vi "Exercise 4.2.vi"() -> ()   [LabVIEW 2010]
panel:
  out "Loop Iterations":i32
  out "Dispense\nChange":bool
  out "Change\nDispensed ($)":dbl format="%.2f"
  out "Vend\nSoda":bool
  out "Money Inserted ($)":dbl format="%.2g"
  in  "Coin to Insert":T1(ring)
  in  "stop":bool
  in  "Insert Coin":bool
  # "All Products in this vending machine cost $0.50"
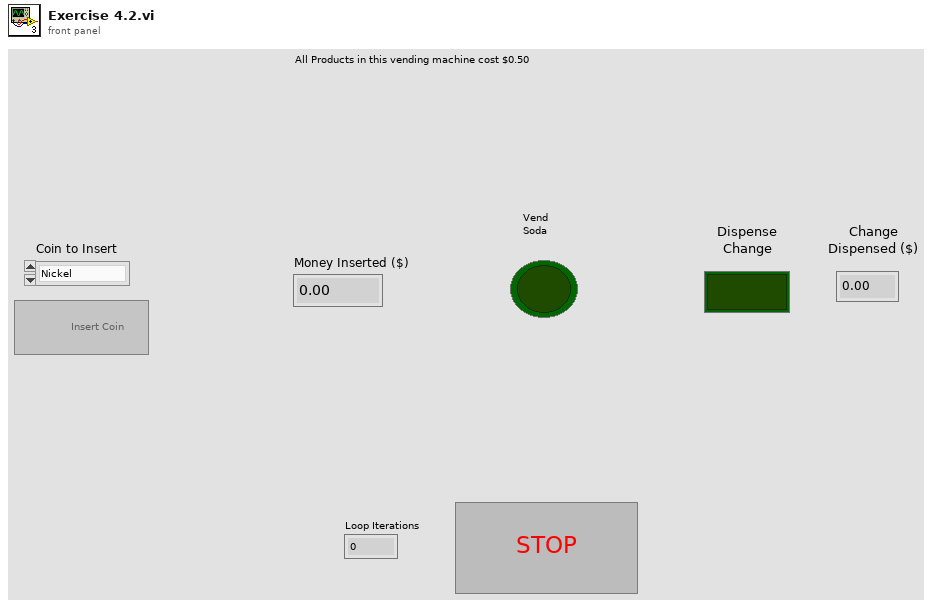
[diagram p1: front panel]
types:
  T1 = enum16{"Nickel", "Dime", "Quarter", "Exit", "Vend", "Change", "Wait", "Initialize"}
  T2 = enum8{"Enabled", "Disabled", "Disabled and Grayed Out"}
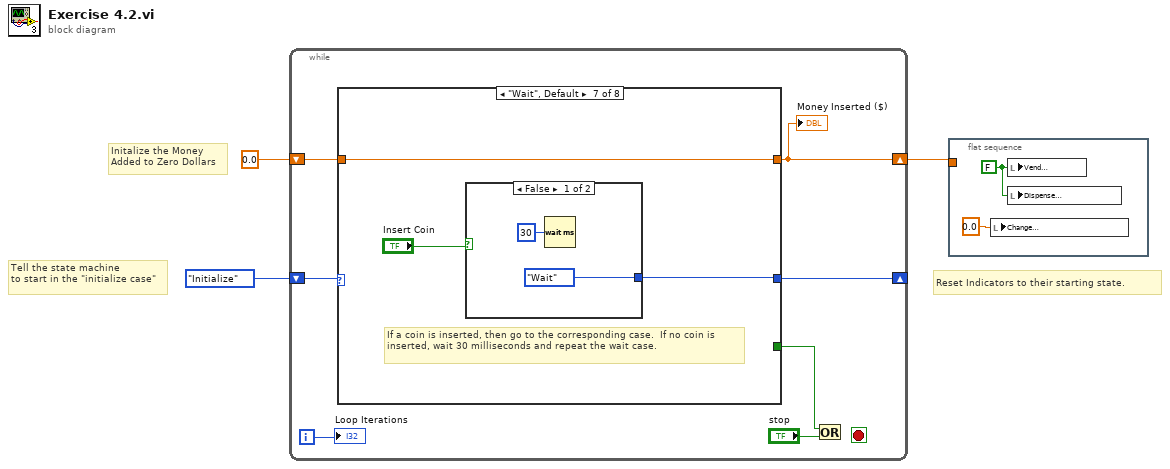
[diagram p0: block diagram]
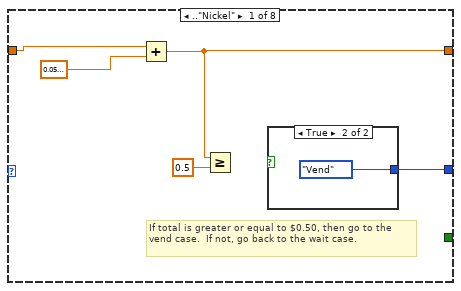
[diagram p2: hidden frame]
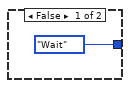
[diagram p3: hidden frame]
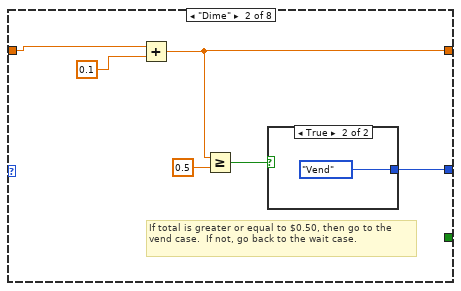
[diagram p4: hidden frame]
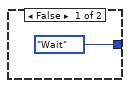
[diagram p5: hidden frame]
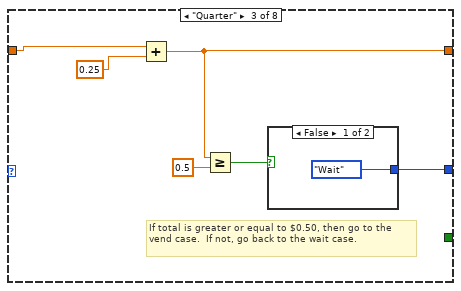
[diagram p6: hidden frame]
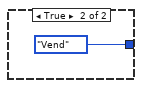
[diagram p7: hidden frame]
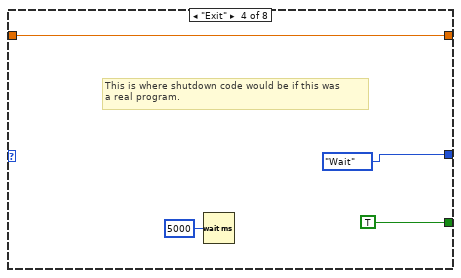
[diagram p8: hidden frame]
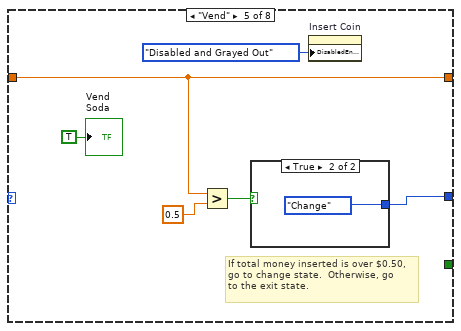
[diagram p9: hidden frame]
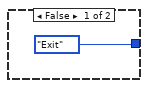
[diagram p10: hidden frame]
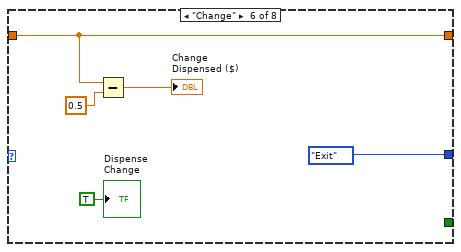
[diagram p11: hidden frame]
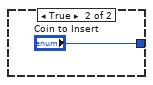
[diagram p12: hidden frame]
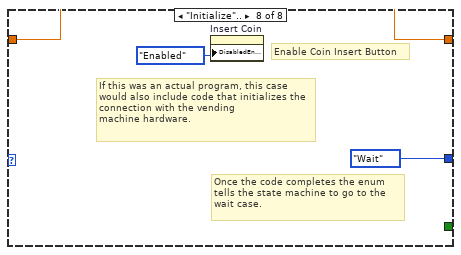
[diagram p13: hidden frame]
diagram:
  # "Reset Indicators to their starting state."
  # "Tell the state machine\nto start in the \"initialize case\""
  # "Initalize the Money\nAdded to Zero Dollars"
  n1 = while {
    shift-right: [w9] -> _
    shift-left: T1."Initialize" -> [w10]
    shift-right: [w7] -> w1
    shift-left: 0.0 -> [w8]
    i -> [w4]
    stop <- _ stop-if-true
    n2 = case shown="\"Wait\", Default" w10 {
      tunnel: [w15 w23 w31 T1."Wait" w43 T1."Exit" w52 T1."Wait"] -> w9
      tunnel: w8 -> [w13 w21 w29 w36 w41 w49 w51 w57]
      tunnel: [w11 w18 w26 w36 w41 w49 w51 w57] -> w7
      tunnel: [_ _ _ TRUE _ _ _ _] -> w5
      frame .."Nickel" {
        # "If total is greater or equal to $0.50, then go to the vend case.  If not, go back to the wait case."
        n3 = Add(x=w13, y=sgl 0.05) -> (x+y=w11:dbl)
        n4 = Greater Or Equal?(x=w11, y=sgl 0.5) -> ()  [unwired: 1 out]
        n5 = case shown="True" {
          selector: _ -> [_ _]
          tunnel: [T1."Wait" T1."Vend"] -> w15
          frame False {
          }
          frame True {
          }
        }
      }
      frame "Dime" {
        # "If total is greater or equal to $0.50, then go to the vend case.  If not, go back to the wait case."
        n6 = Add(x=w21, y=0.1) -> (x+y=w18:dbl)
        n7 = Greater Or Equal?(x=w18, y=sgl 0.5) -> (x >= y?=w19:bool)
        n8 = case shown="True" w19 {
          tunnel: [T1."Wait" T1."Vend"] -> w23
          frame False {
          }
          frame True {
          }
        }
      }
      frame "Quarter" {
        # "If total is greater or equal to $0.50, then go to the vend case.  If not, go back to the wait case."
        n9 = Add(x=w29, y=0.25) -> (x+y=w26:dbl)
        n10 = Greater Or Equal?(x=w26, y=sgl 0.5) -> (x >= y?=w27:bool)
        n11 = case shown="False" w27 {
          tunnel: [T1."Wait" T1."Vend"] -> w31
          frame False {
          }
          frame True {
          }
        }
      }
      frame "Exit" {
        # "This is where shutdown code would be if this was \na real program."
        n12 = Wait (ms)(milliseconds to wait=u32 5000) -> ()  [unwired: 1 out]
      }
      frame "Vend" {
        # "If total money inserted is over $0.50,\ngo to change state.  Otherwise, go\nto the exit state."
        n13 = Greater?(x=w41, y=sgl 0.5) -> (0:w39:bool)
        n14 = case shown="True" w39 {
          tunnel: [T1."Exit" T1."Change"] -> w43
          frame False {
          }
          frame True {
          }
        }
        n15 = property on="Insert Coin" class="Bool"("DisabledEnum"=T2."Disabled and Grayed Out" ("Disabled")) -> ()  [unwired: 2 in, 2 out]
        "Vend\nSoda" <- TRUE ("Vend Soda")
      }
      frame "Change" {
        n16 = Subtract(x=w49, y=0.5) -> (x-y=→"Change\nDispensed ($)":dbl)
        "Dispense\nChange" <- TRUE ("Dispense\nChange")
      }
      frame "Wait", Default {
        # "If a coin is inserted, then go to the corresponding case.  If no coin is inserted, wait 30 milliseconds and repeat the wait case."
        n17 = case shown="False" "Insert Coin" {
          tunnel: [T1."Wait" "Coin to Insert"] -> w52
          frame False {
            n18 = Wait (ms)(milliseconds to wait=u32 30) -> ()  [unwired: 1 out]
          }
          frame True {
          }
        }
      }
      frame "Initialize".. {
        # "Enable Coin Insert Button"
        # "Once the code completes the enum\ntells the state machine to go to the \nwait case."
        # "If this was an actual program, this case would also include code that initializes the connection with the vending\nmachine hardware."
        n19 = property on="Insert Coin" class="Bool"("DisabledEnum"=T2."Enabled" ("Disabled")) -> ()  [unwired: 2 in, 2 out]
      }
    }
    "Money Inserted ($)" <- w7
    n20 = Or(x=w5, y="stop") -> ()  [unwired: 1 out]
    "Loop Iterations" <- w4
  }
  n21 = flat-sequence {
    tunnel: w1 -> [_]
    frame #0 {
      w61 = FALSE ("Dispense\nChange")
      n22 = local write "Change\nDispensed ($)"(0.0 ("Change\nDispensed ($)")) -> ()
      n23 = local write "Vend\nSoda"(w61) -> ()
      n24 = local write "Dispense\nChange"(w61) -> ()
    }
  }
